vi "get_FPGA_ref.vi"(8 "error in":errorcluster) -> (0 "error out":errorcluster, 2 "Is empty?":bool, 3 "FPGA Reference":T1)   [LabVIEW 2010, in "FPGAWrapperRK110909Throughput.lvclass"]
uses:
  FPGAWrapperRK110909Throughput.lvclass
  FPGA_reference.ctl
  class_data.vi
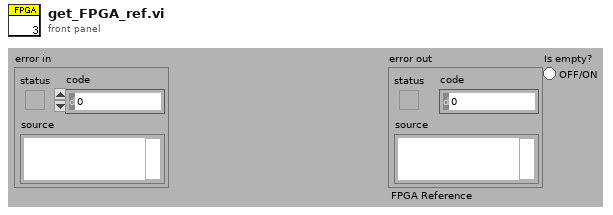
[diagram p1: front panel]
types:
  T1 = typedef "FPGAWrapperRK110909Throughput.lvclass/FPGA_reference.ctl" = refnum<k20>
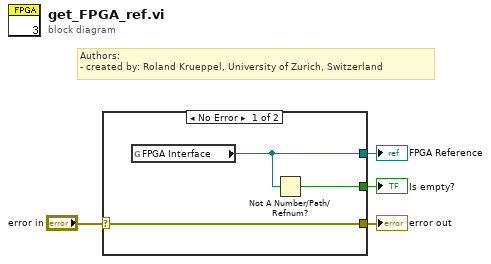
[diagram p0: block diagram]
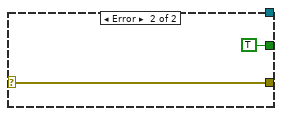
[diagram p2: hidden frame]
diagram:
  # "Authors: \n- created by: Roland Krueppel, University of Zurich, Switzerland"
  n1 = case shown="No Error" "error in" {
    selector: "error in" -> [w7 w9]
    tunnel: [w7 w9] -> w3
    tunnel: [w6 _] -> w2
    tunnel: [w5 TRUE] -> w1
    frame No Error {
      n2 = global read "class_data.vi" "FPGA Interface"() -> (w6:T1)
      n3 = Not A Number/Path/Refnum?(number/path/refnum=w6) -> (NaN/Path/Refnum?=w5:bool)
    }
    frame Error {
    }
  }
  "error out" <- w3
  "FPGA Reference" <- w2
  "Is empty?" <- w1
